vi "Calculate frame rate.vi"() -> (3 "Frame rate (fps)":dbl)   [LabVIEW 2013]
uses:
  Typedefs/Frame Size.ctl
  Global Variables/General Globals.vi
  Global Variables/gl_UI Ctrl Refs.vi
panel:
  in  "Press to enable test inputs":bool
  in  "Dwell time (us)":dbl=0.05 min=0.05 max=12.0 step=0.05
  in  "AOD fill time (us)":dbl=24.4
  in  "Frame size":T1=512 items=["100X100"=100, "128X128"=128, "200X200"=200, "256X256"=256, "512X512"=512, "1024x1024"=1024, "2048x2048"=2048]
  # "Test Inputs"
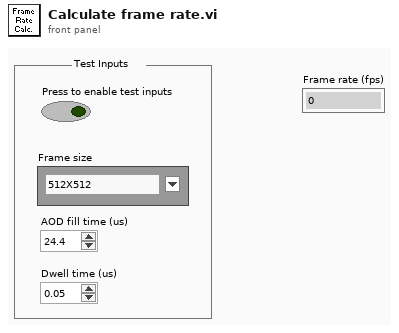
[diagram p1: front panel]
types:
  T1 = typedef "Frame Size.ctl" = u16
  T2 = typedef "Imaging Protocols enum.ctl" = enum16{"AOL Z-Stack", "Motor Z Stack", "Functional Acquisition", "Single Plane Acquisition", "Volume Acquisition", "Live Imaging", "Live Plane Imaging", "Live Volume Imaging"}
  T3 = typedef "UI ctrl refs cluster.ctl" = cluster{"Top level VI path":path, "Top level VI ref":refnum<vi>, "User menu ref":refnum<k9>, "Sub Panel control":refnum<vi>, "Imaging Param Tab":refnum<vi>, "Occurrence-Start drivers":refnum<k4>, "Occurrence-Speed logging initialised":refnum<k4>, "Occurrence-XYZ stage initialised":refnum<k4>, "Exit button":refnum<vi>, "Status ind":refnum<vi>, "Return to Origin":refnum<vi>, "Speed Logging":refnum<vi>, "Time Lapse":refnum<vi>, "Live Imaging":refnum<vi>, "AOL Z Stack":refnum<vi>, "Motor Z Stack":refnum<vi>, "Funct Acq button":refnum<vi>, "Hard Shutter":refnum<vi>, "Virtual Shutter":refnum<vi>, "Laser Power":refnum<vi>, "AOL Mode":refnum<vi>, "Frame Size":refnum<vi>, "Field of View":refnum<vi>, "Dwell Time":refnum<vi>, "Zoom":refnum<vi>, "AOL Z":refnum<vi>, "Objective":refnum<vi>, "Axis":refnum<vi>, "Paths & Names":refnum<vi>, "Experiment folder path (ind.)":refnum<vi>, "Last State (Ind.)":refnum<vi>, "Laser wavelength ind (nm)":refnum<vi>, "Averages":refnum<vi>, "Angle (degrees)":refnum<vi>, "X centre":refnum<vi>, "Y centre":refnum<vi>, "Plane Mode":refnum<vi>, "# Planes":refnum<vi>, "Z Start":refnum<vi>, "Z Stop":refnum<vi>, "Z Step":refnum<vi>, "PMT 1":refnum<vi>, "PMT 2":refnum<vi>, "Stage XYZ Position":refnum<vi>, "Pockels@Z Start":refnum<vi>, "Pockels@Z Stop":refnum<vi>, "Obtain Z Start":refnum<vi>, "Obtain Z Stop":refnum<vi>, "Live stim.trig.period":refnum<vi>, "Live stim.trig.enable":refnum<vi>, "Funct. Acq. Pockels Modulation":refnum<vi>, "Enable Video Recording":refnum<vi>, "Video Record-Live Imaging":refnum<vi>, "Video Record-Funct acq":refnum<vi>, "AOL Z-stack Chirps Ready (ind)":refnum<vi>, "Center freq ind (nm)":refnum<vi>, "Logging queue (ind)":refnum<vi>, "Back aperture power (ind.)":refnum<vi>, "Power after objective (ind.)":refnum<vi>, "Switch user":refnum<vi>}
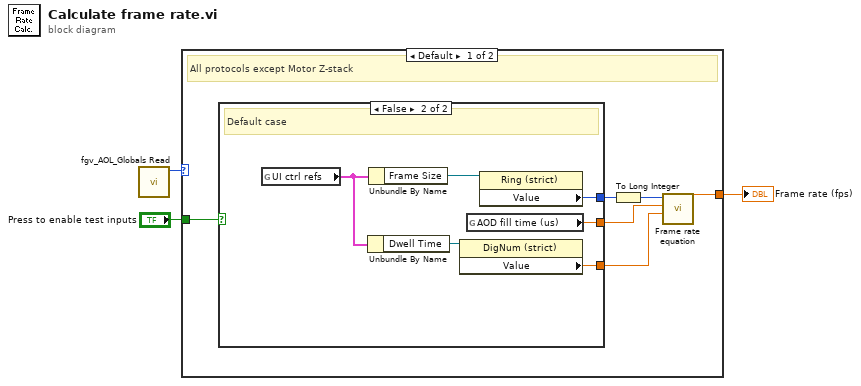
[diagram p0: block diagram]
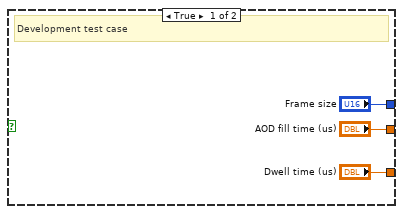
[diagram p2: hidden frame]
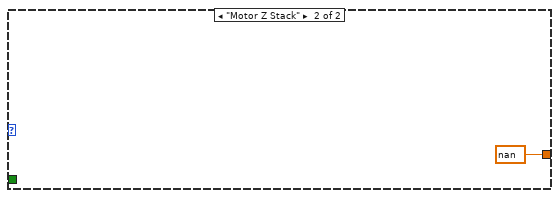
[diagram p3: hidden frame]
diagram:
  n1 = call "fgv_AOL_Globals Read.vi"() -> ("Imaging Protocol"=w1:T2)  [unwired: 9 in, 2 out]
  n2 = case shown="Default" w1 {
    tunnel: [w9 nan ("FrameRate (fps)")] -> w3
    tunnel: "Press to enable test inputs" -> [w4 _]
    frame Default {
      # "All protocols except Motor Z-stack"
      n3 = case shown="False" w4 {
        tunnel: ["Dwell time (us)" w18] -> w8
        tunnel: ["AOD fill time (us)" w17] -> w7
        tunnel: ["Frame size" w16] -> w6
        frame True {
          # "Development test case"
        }
        frame False {
          # "Default case"
          n4 = global read "gl_UI Ctrl Refs.vi" "UI ctrl refs"() -> (w15:T3)
          n5 = Unbundle By Name(w15) -> ("Dwell Time"=w14:refnum<vi>)
          n6 = Unbundle By Name(w15) -> ("Frame Size"=w13:refnum<vi>)
          n7 = property on="Property Node" class="DigNum (strict)"(reference=w14) -> ("Value"=w18:dbl)  [unwired: 1 in, 2 out]
          n8 = global read "General Globals.vi" "AOD fill time (us)"() -> (w17:dbl)
          n9 = property on="Property Node" class="Ring (strict)"(reference=w13) -> ("Value"=w16:T1)  [unwired: 1 in, 2 out]
        }
      }
      n10 = To Long Integer(number=w6) -> (32bit integer=w5:i32)
      n11 = call "Frame rate equation.vi"("Dwell time (us)"=w8, "AOD fill time (us)"=w7, "Frame size (single dimension)"=w5) -> ("FrameRate (fps)"=w9:dbl)  [unwired: 8 in]
    }
    frame "Motor Z Stack" {
    }
  }
  "Frame rate (fps)" <- w3
